vi "StationInfo@SetStationON__Parameter.vi"(1 "ParamterIn":string) -> (0 "ParamterOut":string)   [LabVIEW 2020]
uses:
  CoreModules/StationModule/StationData.ctl
panel:
  in  "StationName":string(combo)
  in  "Confirm":bool
  # "StationInfo@SetStationON $Station"
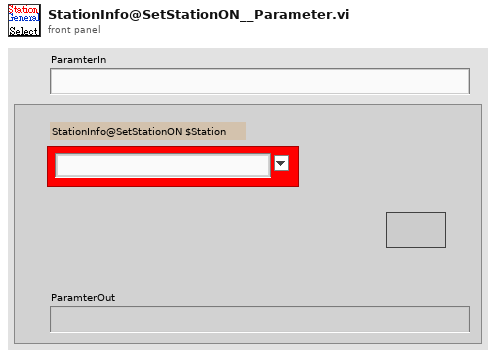
[diagram p1: front panel]
types:
  T1 = typedef "StationData.ctl" = enum16{"ResetDefault", "SetStationOK", "SetStationNG", "UpdateIndicator", "GetData", "SetData", "StateShift", "Init", "SetStationON", "SetStationOFF", "BlinkingON", "BlinkingOFF"}
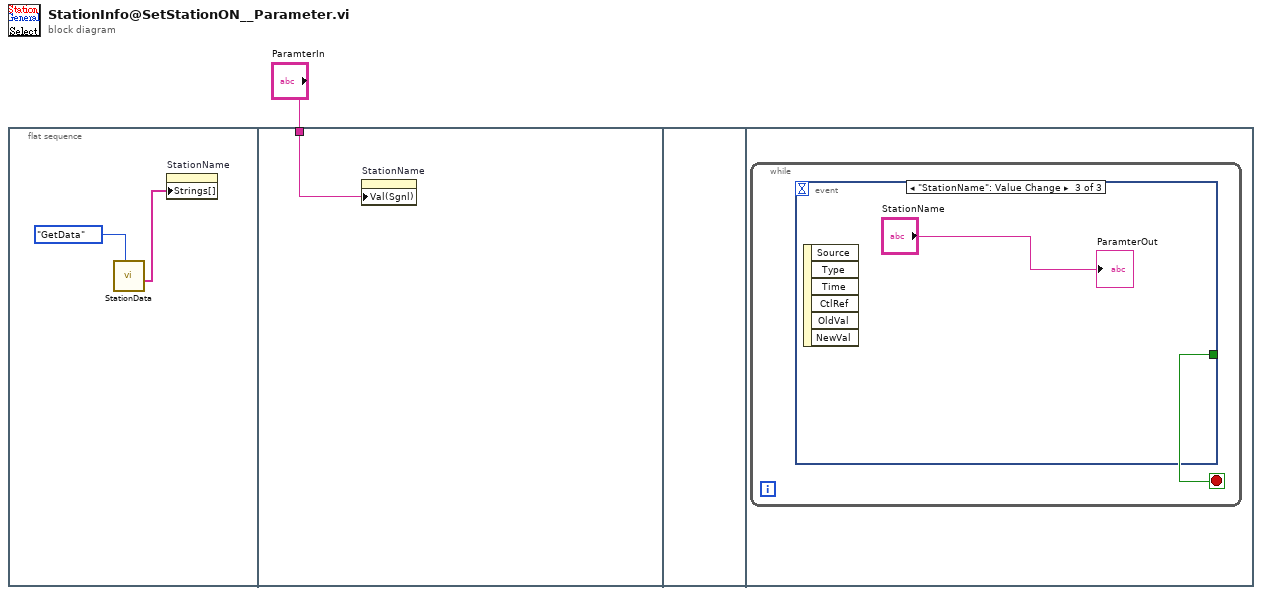
[diagram p0: block diagram]
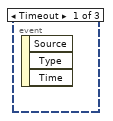
[diagram p2: hidden frame]
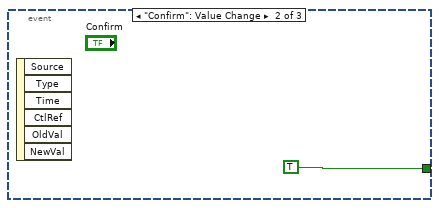
[diagram p3: hidden frame]
diagram:
  n1 = flat-sequence {
    tunnel: "ParamterIn" -> [w4]
    frame #0 {
      n2 = call "StationData.vi"("CMD"=StationData."GetData") -> ("StationList"=w2:string[])  [unwired: 8 in, 2 out]
      n3 = property on="StationName" class="CmbBox"("Strings[]"=w2) -> ()  [unwired: 2 in, 2 out]
    }
    frame #1 {
      n4 = property on="StationName" class="CmbBox"("Val(Sgnl)"=w4) -> ()  [unwired: 2 in, 2 out]
    }
    frame #2 {
    }
    frame #3 {
      n5 = while {
        stop <- w5 stop-if-true
        n6 = event shown="[2] \"StationName\": Value Change" {
          selector: _ -> [_ _ _]
          dyn-events: _ -> [_ _ _]
          timeout: _ -> [_ _ _]
          tunnel: [_ TRUE _] -> w5
          event Timeout {
            n7 = event-data() -> ()  [unwired: 1 in, 3 out]
          }
          event "Confirm": Value Change {
            n8 = event-data() -> ()  [unwired: 1 in, 6 out]
          }
          event "StationName": Value Change {
            n9 = event-data() -> ()  [unwired: 1 in, 6 out]
            "ParamterOut" <- "StationName"
          }
        }
      }
    }
  }
